vi "Clear.vi"(3 "(WavIndex_Pointer) in":refnum<class "WavIndex_Pointer.lvclass">) -> (1 "(WavIndex_Pointer) out":refnum<class "WavIndex_Pointer.lvclass">)   [LabVIEW 2020, in "WavIndex_Pointer.lvclass"]
uses:
  WavIndex_Pointer.lvclass
  WavIndex_Pointer.lvclass/WavIndex_Pointer.ctl
  Index_Pointer/Index_Pointer.lvclass
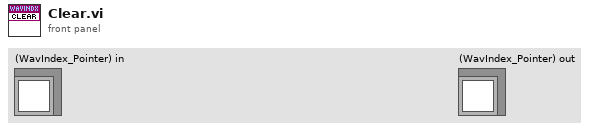
[diagram p1: front panel]
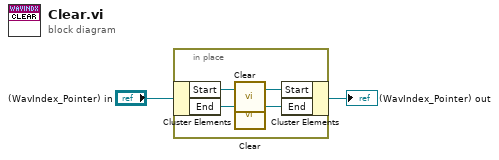
[diagram p0: block diagram]
diagram:
  n1 = in-place {
    n2 = in-place-cluster #1("(WavIndex_Pointer) in") -> ("Start"=w6:refnum<class "Index_Pointer.lvclass">, "End"=w5:refnum<class "Index_Pointer.lvclass">)
    n3 = call-dynamic "Clear.vi"("(Index_Pointer) in"=w6) -> ("(Index_Pointer) out"=w3:refnum<class "Index_Pointer.lvclass">)  [unwired: 2 in]
    n4 = call-dynamic "Clear.vi"("(Index_Pointer) in"=w5) -> ("(Index_Pointer) out"=w4:refnum<class "Index_Pointer.lvclass">)  [unwired: 2 in]
    n5 = in-place-cluster #1("Start"=w3, "End"=w4) -> (→"(WavIndex_Pointer) out":refnum<class "WavIndex_Pointer.lvclass">)
  }
